vi "ImageOverlay.vi"(11 "Refnum in":T1) -> (3 "Refnum out":T1)   [LabVIEW 2014]
uses:
  <vilib>/vision/Image Controls.llb/IMAQ Image.ctl
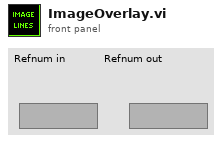
[diagram p1: front panel]
types:
  T1 = typedef "IMAQ Image.ctl" = refnum<image>
  T2 = cluster{"Left":i32, "Top":i32, "Right":i32, "Bottom":i32}
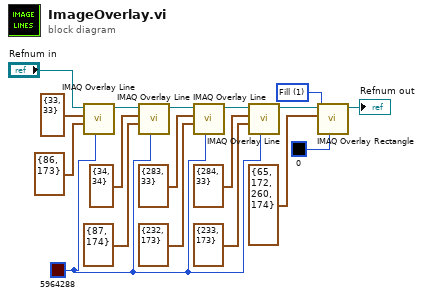
[diagram p0: block diagram]
diagram:
  w1 = u32 1 items=["Frame", "Fill", "Highlight"] ("Drawing Mode (Frame)")
  w6 = u32 5964288 ("Color")
  n1 = call "IMAQ Overlay Line"("Color"=w6, "End Point"=cluster{"X":i32, "Y":i32} {"X"=86, "Y"=173}, "Start Point"=cluster{"X":i32, "Y":i32} {"X"=33, "Y"=33}, "Image"="Refnum in") -> ("Image Out"=w16:T1)  [unwired: 6 in, 1 out]
  n2 = call "IMAQ Overlay Line"("Color"=w6, "End Point"=cluster{"X":i32, "Y":i32} {"X"=87, "Y"=174}, "Start Point"=cluster{"X":i32, "Y":i32} {"X"=34, "Y"=34}, "Image"=w16) -> ("Image Out"=w8:T1)  [unwired: 6 in, 1 out]
  n3 = call "IMAQ Overlay Line"("Color"=w6, "End Point"=cluster{"X":i32, "Y":i32} {"X"=232, "Y"=173}, "Start Point"=cluster{"X":i32, "Y":i32} {"X"=283, "Y"=33}, "Image"=w8) -> ("Image Out"=w7:T1)  [unwired: 6 in, 1 out]
  n4 = call "IMAQ Overlay Line"("Color"=w6, "End Point"=cluster{"X":i32, "Y":i32} {"X"=233, "Y"=173}, "Start Point"=cluster{"X":i32, "Y":i32} {"X"=284, "Y"=33}, "Image"=w7) -> ("Image Out"=w5:T1)  [unwired: 6 in, 1 out]
  n5 = call "IMAQ Overlay Rectangle"("Color"=u32 0, "Drawing Mode (Frame)"=w1, "Rectangle"=T2 {"Left"=65, "Top"=172, "Right"=260, "Bottom"=174}, "Image"=w5) -> ("Image Out"=→"Refnum out":T1)  [unwired: 6 in, 1 out]
